vi "Runvi.vi"(1 "状态":T1(ring)=enum."Standard", 2 "名称或相对路径":string) -> ()   [LabVIEW 2018]
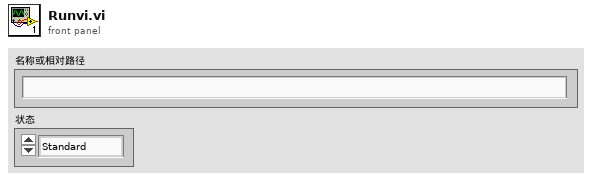
[diagram p1: front panel]
types:
  T1 = enum32{"Invalid", "Standard", "Closed", "Hidden", "Minimized", "Maximized"}
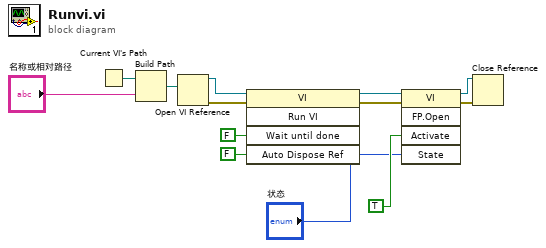
[diagram p0: block diagram]
diagram:
  n1 = Current VI's Path() -> (path=w13:path)
  n2 = Build Path(base path=w13, name or relative path="名称或相对路径") -> (appended path=w12:path)
  n3 = Open VI Reference(vi path=w12) -> (vi reference=w11:refnum<vi>, error out=w10:errorcluster)  [unwired: 5 in]
  n4 = invoke class="VI" method="Run VI"(reference=w11, error in=w10, "Wait until done"=FALSE ("Wait Until Done"), "Auto Dispose Ref"=FALSE ("Auto Dispose Reference")) -> (reference out=w6:refnum<vi>, error out=w7:errorcluster)  [unwired: 1 in, 3 out]
  n5 = invoke class="VI" method="FP.Open"(reference=w6, error in=w7, "Activate"=TRUE ("Activate?"), "State"="状态") -> (reference out=w3:refnum<vi>, error out=w4:errorcluster)  [unwired: 1 in, 3 out]
  n6 = Close Reference(reference=w3, error in (no error)=w4) -> ()  [unwired: 1 out]
